vi "FGV SGSF und SGSO weiterleiten.vi"(0 "AGSF":string[](array[string]), 1 "SGSF":string[](array[string]), 7 "AGSO":string[](array[string]), 9 "SGSO":string[](array[string]), 11 "error in (no error)":errorcluster caption="Fehler (Eingang, kein Fehler)", 13 "Aktion":T1) -> (2 "SGSF aktuell":bool, 3 "SGSF":string, 4 "AGSF":string, 6 "AGSF aktuell":bool, 8 "AGSO":string, 10 "AGSO aktuell":bool, 12 "SGSO aktuell":bool, 14 "SGSO":string, 15 "error out":errorcluster caption="Fehler (Ausgang)")   [LabVIEW 2020, in "FT-IR.lvlib" / "Spanfaktor.lvlib"]
uses:
  Spanfaktor.lvlib
  Aktion FGV SGSF und SGSO weiterleiten.ctl
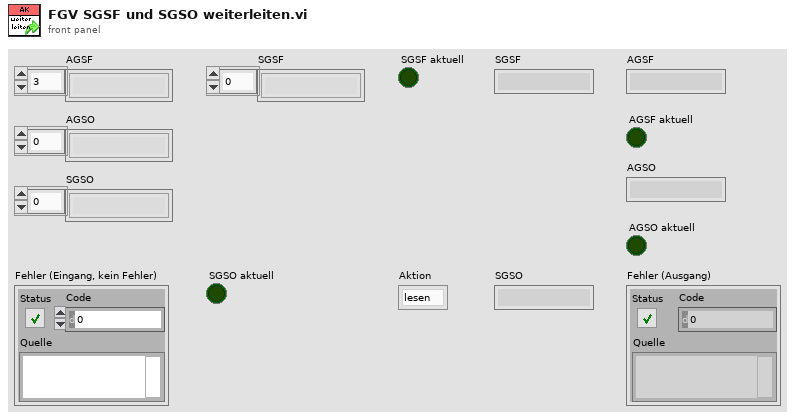
[diagram p1: front panel]
types:
  T1 = typedef "FT-IR.lvlib/Spanfaktor.lvlib/Aktion FGV SGSF und SGSO weiterleiten.ctl" = enum16{"lesen", "AGSF", "AGSO", "AGSF löschen", "AGSO löschen", "SGSF", "SGSO", "SGSF löschen", "SGSO löschen"}
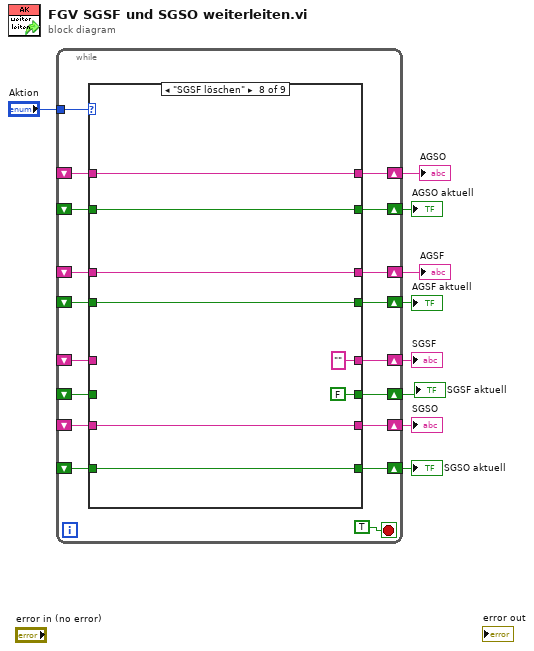
[diagram p0: block diagram]
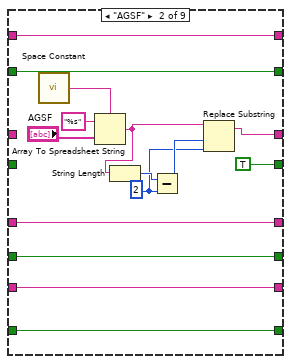
[diagram p3: hidden frame]
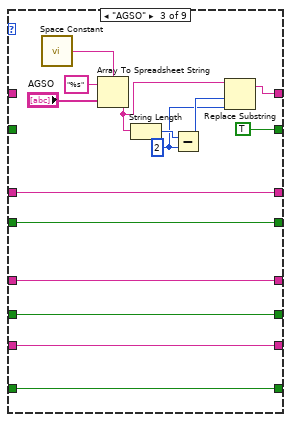
[diagram p4: hidden frame]
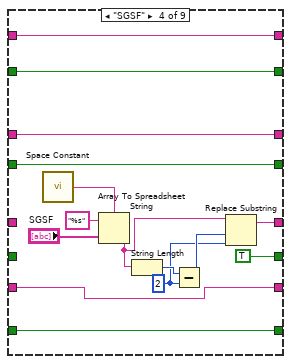
[diagram p5: hidden frame]
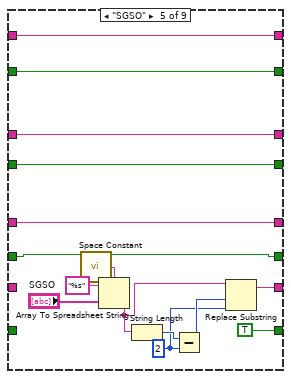
[diagram p6: hidden frame]
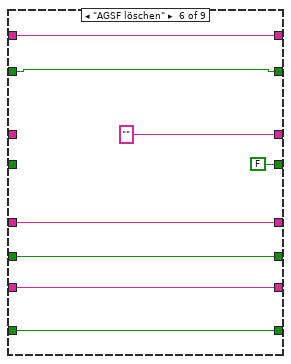
[diagram p7: hidden frame]
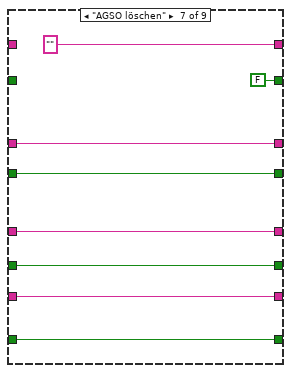
[diagram p8: hidden frame]
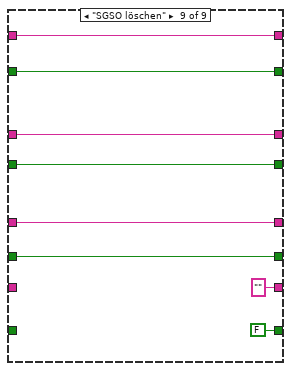
[diagram p9: hidden frame]
diagram:
  n1 = while {
    tunnel: "Aktion" -> [w26]
    shift-right: [w25] -> w8
    shift-left: _ -> [w24]
    shift-right: [w23] -> w7
    shift-left: _ -> [w22]
    shift-right: [w21] -> w6
    shift-left: _ -> [w20]
    shift-right: [w19] -> w5
    shift-left: _ -> [w18]
    shift-right: [w17] -> w4
    shift-left: _ -> [w16]
    shift-right: [w15] -> w3
    shift-left: _ -> [w14]
    shift-right: [w13] -> w1
    shift-left: _ -> [w12]
    shift-right: [w11] -> w2
    shift-left: _ -> [w10]
    stop <- TRUE stop-if-true
    n2 = case shown="\"SGSF löschen\"" w26 {
      tunnel: [w35 w40 w65 w80 w95 "" ("SGSF") w111 w119 w127] -> w25
      tunnel: w24 -> [w35 _ w65 w80 w95 _ w111 w119 w127]
      tunnel: [w34 w50 w55 w70 w86 w103 "" ("SGSO") w118 w126] -> w23
      tunnel: w22 -> [w34 w50 _ w70 w86 w103 _ w118 w126]
      tunnel: [w33 TRUE w61 w76 w91 FALSE w109 w117 w125] -> w21
      tunnel: w20 -> [w33 _ w61 w76 w91 _ w109 w117 w125]
      tunnel: [w32 w45 TRUE w68 w83 w100 FALSE w116 w124] -> w19
      tunnel: w18 -> [w32 w45 _ w68 w83 w100 _ w116 w124]
      tunnel: [w31 w39 w54 w71 w85 w99 w107 "" ("result string") w123] -> w17
      tunnel: w16 -> [w31 w39 w54 _ w85 w99 w107 _ w123]
      tunnel: [w30 w38 w53 w69 w84 w98 w106 w115 "" ("result string")] -> w15
      tunnel: w14 -> [w30 w38 w53 w69 _ w98 w106 w115 _]
      tunnel: [w29 w37 w52 TRUE w82 w97 w105 FALSE w121] -> w13
      tunnel: w12 -> [w29 w37 w52 _ w82 w97 w105 _ w121]
      tunnel: [w28 w36 w51 w66 TRUE w96 w104 w112 FALSE] -> w11
      tunnel: w10 -> [w28 w36 w51 w66 _ w96 w104 w112 _]
      frame "lesen", Default {
      }
      frame "AGSF" {
        w42 = 2 ("y")
        n3 = call <vilib>:"Space Constant.vi"() -> ("String"=w49:string)
        n4 = Array To Spreadsheet String(delimiter (Tab)=w49, array="AGSF", 3:"%s" ("Format-String")) -> (spreadsheet string=w41:string)
        n5 = String Length(string=w41) -> (length=w44:i32)
        n6 = Subtract(x=w44, y=w42) -> (x-y=w43:i32)
        n7 = Replace Substring(2:w42, 3:w43, 5:w41) -> (1:w40:string)  [unwired: 1 in, 1 out]
      }
      frame "AGSO" {
        w57 = 2 ("y")
        n8 = call <vilib>:"Space Constant.vi"() -> ("String"=w63:string)
        n9 = Array To Spreadsheet String(delimiter (Tab)=w63, array="AGSO", 3:"%s" ("Format-String")) -> (spreadsheet string=w56:string)
        n10 = String Length(string=w56) -> (length=w59:i32)
        n11 = Subtract(x=w59, y=w57) -> (x-y=w58:i32)
        n12 = Replace Substring(2:w57, 3:w58, 5:w56) -> (1:w55:string)  [unwired: 1 in, 1 out]
      }
      frame "SGSF" {
        w73 = 2 ("y")
        n13 = call <vilib>:"Space Constant.vi"() -> ("String"=w78:string)
        n14 = Array To Spreadsheet String(delimiter (Tab)=w78, array="SGSF", 3:"%s" ("Format-String")) -> (spreadsheet string=w72:string)
        n15 = String Length(string=w72) -> (length=w75:i32)
        n16 = Subtract(x=w75, y=w73) -> (x-y=w74:i32)
        n17 = Replace Substring(2:w73, 3:w74, 5:w72) -> (1:w71:string)  [unwired: 1 in, 1 out]
      }
      frame "SGSO" {
        w88 = 2 ("y")
        n18 = call <vilib>:"Space Constant.vi"() -> ("String"=w93:string)
        n19 = Array To Spreadsheet String(delimiter (Tab)=w93, array="SGSO", 3:"%s" ("Format-String")) -> (spreadsheet string=w87:string)
        n20 = String Length(string=w87) -> (length=w90:i32)
        n21 = Subtract(x=w90, y=w88) -> (x-y=w89:i32)
        n22 = Replace Substring(2:w88, 3:w89, 5:w87) -> (1:w84:string)  [unwired: 1 in, 1 out]
      }
      frame "AGSF löschen" {
      }
      frame "AGSO löschen" {
      }
      frame "SGSF löschen" {
      }
      frame "SGSO löschen" {
      }
    }
  }
  "AGSF" <- w8
  "AGSO" <- w7
  "AGSF aktuell" <- w6
  "AGSO aktuell" <- w5
  "SGSF" <- w4
  "SGSO" <- w3
  "SGSO aktuell" <- w2
  "SGSF aktuell" <- w1
